vi "240124_Init-PI_E709.vi"(8 "error in (no error)":errorcluster) -> (0 "error out":errorcluster, 3 "E-709-cluster":T1)   [LabVIEW 2014]
doc: "This VI is used to initialize the XY stage (E-709).\nIt:\n- starts the communication on the USB port\n- starts to reference the axis\n- sets servo ON and validates this\n- get the current name of the axis\n- get the current positions of the stage\n- get the range of the axis\n*****************************************************************************************\nAttention: il y a une erreur dans le VI de chez PI: RS232 DaisyChain correspond a USB!"
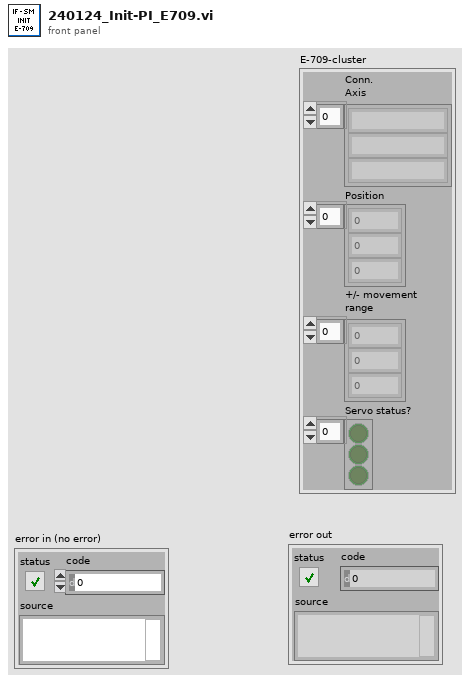
[diagram p1: front panel]
types:
  T1 = cluster{"Conn. \nAxis":string[], "Position":dbl[], "+/- movement\nrange":dbl[], "Servo status?":bool[]}
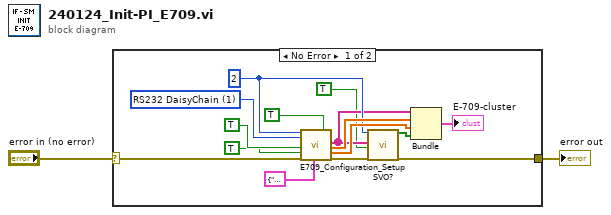
[diagram p0: block diagram]
diagram:
  n1 = case shown="No Error" "error in (no error)" {
    selector: "error in (no error)" -> [w17 w18]
    tunnel: [w11 w18] -> w1
    frame No Error {
      w15 = u16 1 items=["RS232", "RS232 DaisyChain", "USB"] ("Interface")
      w10 = 2 ("System no.")
      n2 = call "E709_Configuration_Setup.vi"("System no."=w10, "Interface"=w15, "Change servo status to ON?"=TRUE, "Perform autozero?"=TRUE, "error in"=w17, "USB settings"=cluster{"S/N":string, "USB Search?":bool} {"S/N"="0115044415", "USB Search?"=TRUE}, "Move to middle?"=TRUE) -> ("Conn. \nAxis"=w9:string[], "Position"=w14:dbl[], "+/- movement\nrange"=w13:dbl[], "error out"=w12:errorcluster)  [unwired: 7 in, 2 out]
      n3 = call "SVO?.vi"("System no."=w10, "Axes to query"=w9, "All axes?"=TRUE, "error in"=w12) -> ("Servo status?"=w7:bool[], "error out"=w11:errorcluster)  [unwired: 14 in]
      n4 = Bundle("Conn. \nAxis"=w9, "Position"=w14, "+/- movement\nrange"=w13, "Servo status?"=w7) -> (→"E-709-cluster":T1)  [unwired: 1 in]
    }
    frame Error {
    }
  }
  "error out" <- w1
